vi "GDSLvIcon_ConvertBoolToColorPicture.vi"(1 "CharPicture":bool[][](array[boolean]), 5 "error in (no error)":errorcluster, 6 "Background color":u32(colorbox)=16777215, 8 "Foreground color":u32(colorbox)) -> (15 "CharPicture out":u8[][](array[numeric]), 19 "error out":errorcluster)   [LabVIEW 2016]
doc: "Applies a text in the upper part of the picture."
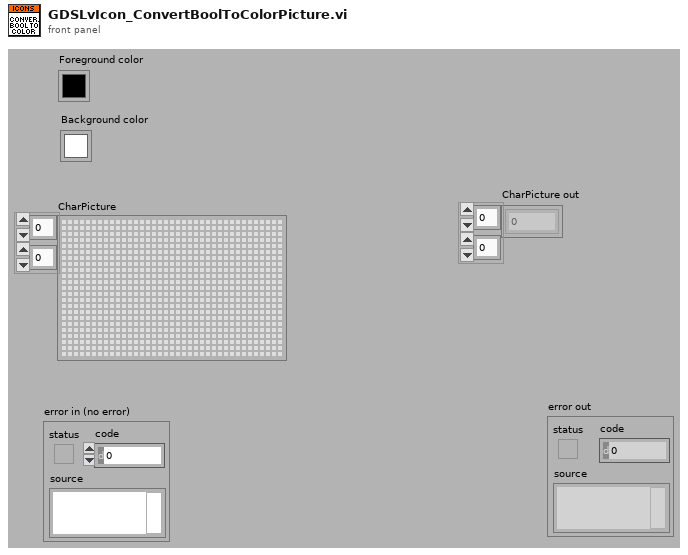
[diagram p1: front panel]
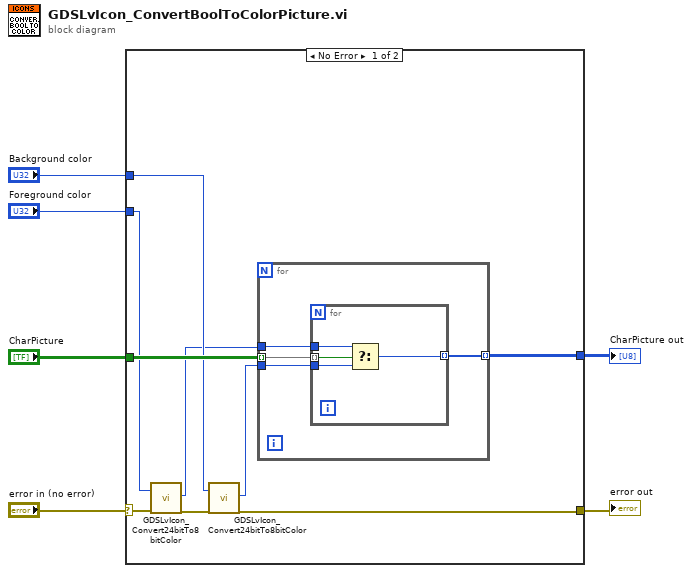
[diagram p0: block diagram]
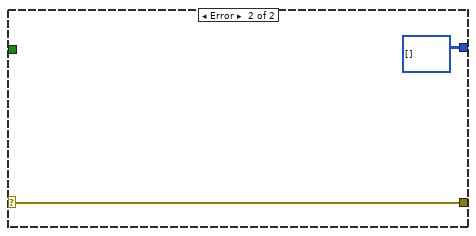
[diagram p2: hidden frame]
diagram:
  n1 = case shown="No Error" "error in (no error)" {
    selector: "error in (no error)" -> [w9 w25]
    tunnel: [w7 w25] -> w5
    tunnel: "Foreground color" -> [w12 _]
    tunnel: "Background color" -> [w13 _]
    tunnel: "CharPicture" -> [w15 _]
    tunnel: [w14 u8[][] []] -> w1
    frame No Error {
      n2 = call <resource>:"GDSLvIcon_Convert24bitTo8bitColor.vi"("Color 24bit In"=w12, "error in (no error)"=w9) -> ("Color out(256)"=w11:u8, "error out"=w8:errorcluster)  [unwired: 14 in, 2 out]
      n3 = call <resource>:"GDSLvIcon_Convert24bitTo8bitColor.vi"("Color 24bit In"=w13, "error in (no error)"=w8) -> ("Color out(256)"=w10:u8, "error out"=w7:errorcluster)  [unwired: 14 in, 2 out]
      n4 = for {
        tunnel: w15 -> [w19] mode=indexing
        tunnel: w11 -> [w18]
        tunnel: w10 -> [w17]
        tunnel: [w16] -> w14 mode=indexing
        n5 = for {
          tunnel: w19 -> [w23] mode=indexing
          tunnel: w18 -> [w22]
          tunnel: w17 -> [w21]
          tunnel: [w20] -> w16 mode=indexing
          n6 = Select(t=w22, s=w23, f=w21) -> (s? t:f=w20:u8)
        }
      }
    }
    frame Error {
    }
  }
  "error out" <- w5
  "CharPicture out" <- w1
